vi "FUG_PowerSupply.UpdateSign.vi"(0 "i ref in":refnum<vi>, 1 "badValue":bool, 2 "moduleValue":dbl format="%.2f", 3 "ms timeout (10000)":i32=10000, 5 "error in (no error)":errorcluster) -> (14 "i ref out":refnum<vi>, 17 "timed out":bool, 19 "error out":errorcluster)   [LabVIEW 2014, in "FUG_PowerSupply.lvlib"]
doc: "Takes the value published by the module and updates the sign value in the attribute data."
uses:
  FUG_PowerSupply.lvlib
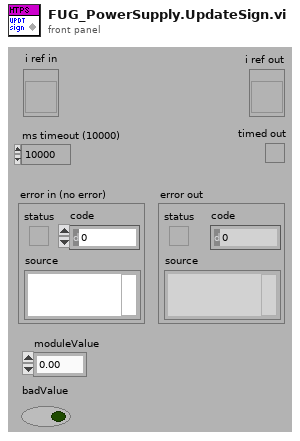
[diagram p1: front panel]
types:
  T1 = typedef "FUG_PowerSupply.lvlib/FUG_PowerSupply.i attribute.ctl" = cluster{"Type":string, "Elektrode Name":string, "CALC_FACTOR_SET_VOLTAGE":dbl, "CALC_FACTOR_GET_VOLTAGE":dbl, "CALC_FACTOR_GET_CURRENT":dbl, "CALC_FACTOR_SET_CURRENT ":dbl, "REG_VALUE":dbl, "Sign":bool, "setVoltID":i32, "setCurrentID":i32, "setPowerOnID":i32, "MaxVoltage":dbl}
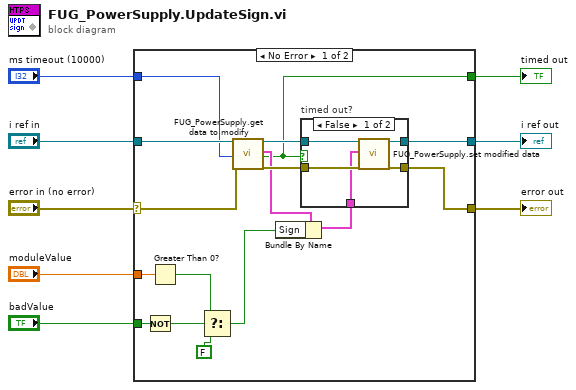
[diagram p0: block diagram]
diagram:
  n1 = case shown="No Error" "error in (no error)" {
    selector: "error in (no error)" -> [w13 w32]
    tunnel: "i ref in" -> [w14 w33]
    tunnel: "moduleValue" -> [w22 _]
    tunnel: "ms timeout (10000)" -> [w10 _]
    tunnel: [w12 w33] -> w5
    tunnel: [w11 w32] -> w4
    tunnel: "badValue" -> [w24 _]
    tunnel: [w9 _] -> w1
    frame No Error {
      n2 = Not(x=w24) -> (.not. x?=w23:bool)
      n3 = Greater Than 0?(x=w22) -> (x > 0?=w21:bool)
      n4 = Select(t=w21, s=w23, f=FALSE) -> (s? t:f=w15:bool)
      n5 = call "FUG_PowerSupply.get data to modify.vi"("i ref in"=w14, "ms timeout (10000)"=w10, "error in (no error)"=w13) -> ("i ref out"=w19:refnum<vi>, "i attribute"=w17:T1, "timed out"=w9:bool, "error out"=w18:errorcluster)  [unwired: 13 in]
      n6 = Bundle By Name(cluster=w17, "Sign"=w15) -> (w16:T1)
      n7 = case "timed out?" shown="False" w9 {
        tunnel: w19 -> [w29 w31]
        tunnel: w18 -> [w28 w30]
        tunnel: [w27 w30] -> w11
        tunnel: [w26 w31] -> w12
        tunnel: w16 -> [w25 _]
        frame False {
          n8 = call "FUG_PowerSupply.set modified data.vi"("i ref in"=w29, "i attribute"=w25, "error in (no error)"=w28) -> ("i ref out"=w26:refnum<vi>, "error out"=w27:errorcluster)  [unwired: 15 in]
        }
        frame True {
        }
      }
    }
    frame Error {
    }
  }
  "error out" <- w4
  "i ref out" <- w5
  "timed out" <- w1
